vi "LED-Set Text_Tag.vi"() -> (4 "\"Set Text\" Label":string)   [LabVIEW 2012, in "LED Display.xctl"]
doc: "This VI sets the tag to \"SetTxt\" with no ability to modify the value of the string when translating to another language."
uses:
  LED Display.xctl
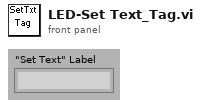
[diagram p1: front panel]
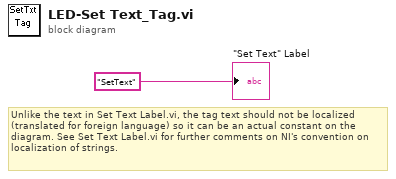
[diagram p0: block diagram]
diagram:
  # "Unlike the text in Set Text Label.vi, the tag text should not be localized (translated for foreign language) so it can be an actual constant on the diagram. See Set Text Label.vi for further comments on NI's convention on localization of strings."
  "\"Set Text\" Label" <- "SetText" ("String")
